vi "19.9-PtByPt and Array Based Filter.vi"() -> ()   [LabVIEW 2020]
doc: "Compares Point By Point filters with array-based filters. The Point By Point filter works in real-time and online while the array-based filter waits for the array to be compiled first. Array-based filter is also called block filter."
uses:
  <vilib>/Analysis/3filter.llb/IIR Filter (DBL).vi
  <vilib>/ptbypt/NI_PtbyPt.lvlib
  <vilib>/Analysis/NI_AALBase.lvlib
panel:
  in  "type":enum16{"moving average", "exponential"}(ring)=enum."exponential"
  out "Graph: Filtered (Array Based)":dbl[](graph)
  out "Chart: Noise Signal":cluster{dbl, "uniform white noise":dbl}(graph)
  in  "Noise level":dbl(slide)=0.2 step=0.05 scale=0.0..5.0
  in  "Initialize Array-based filter":bool
  in  "Stop":bool
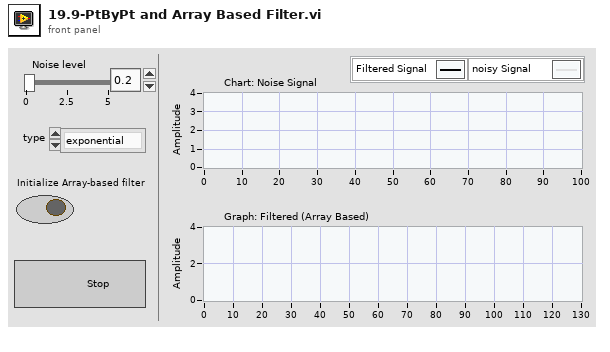
[diagram p1: front panel]
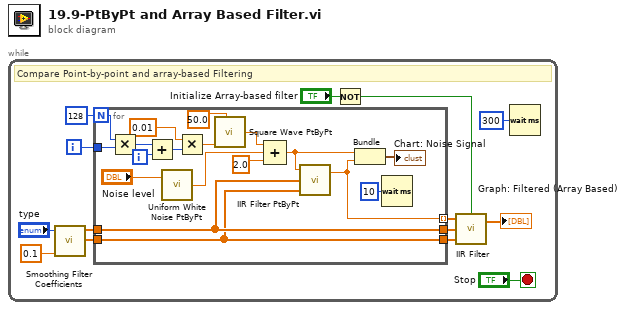
[diagram p0: block diagram]
diagram:
  n1 = while {
    i -> [w13]
    stop <- "Stop" stop-if-true
    # "Compare Point-by-point and array-based Filtering"
    n2 = call <vilib>:"Smoothing Filter Coefficients.vi"("time constant"=0.1, "type"="type") -> ("forward coefficients"=w8:dbl[], "reverse coefficients"=w7:dbl[])  [unwired: 7 in, 1 out]
    n3 = for {
      N: 128 -> [w30]
      tunnel: [w17] -> w2 mode=indexing
      tunnel: w13 -> [w29]
      tunnel: w8 -> [w15]
      tunnel: w7 -> [w16]
      tunnel: [w16] -> w5
      tunnel: [w15] -> w4
      i -> [w32]
      # "Generate signal and filter every point."
      n4 = Multiply(x=w30, y=w29) -> (x*y=w28:i32)
      n5 = Add(x=w28, y=w32) -> (x+y=w25:i32)
      n6 = call <vilib>:"Uniform White Noise PtByPt.vi"("amplitude"="Noise level") -> ("uniform white noise"=w21:dbl)  [unwired: 2 in]
      n7 = Multiply(x=0.01, y=w25) -> (x*y=w23:dbl)
      n8 = call <vilib>:"Square Wave PtByPt.vi"("time"=w23, "duty cycle (%)"=50.0) -> ("square wave"=w19:dbl)  [unwired: 3 in]
      n9 = Compound Arithmetic op=ADD(w19, w21, 2.0) -> (w18:dbl)
      n10 = call <vilib>:"IIR Filter PtByPt.vi"("Forward Coefficients"=w15, "Reverse Coefficients"=w16, "x"=w18) -> ("Filtered x"=w17:dbl)  [unwired: 1 in, 1 out]
      n11 = Bundle(w18, "Filtered x"=w17) -> (→"Chart: Noise Signal":cluster{dbl, "Filtered x":dbl})  [unwired: 1 in]
      n12 = Wait (ms)(milliseconds to wait=u32 10) -> ()  [unwired: 1 out]
    }
    n13 = Not(x="Initialize Array-based filter") -> (.not. x?=w6:bool)
    n14 = call-poly <vilib>:"IIR Filter.vi"("init/cont (init:F)"=w6, "Forward Coefficients"=w4, "Reverse Coefficients"=w5, "X"=w2) -> ("Filtered X"=→"Graph: Filtered (Array Based)":dbl[])  [unwired: 1 out]
    n15 = Wait (ms)(milliseconds to wait=u32 300) -> ()  [unwired: 1 out]
  }
